vi "Write Param.vi"(0 "PID SP Limiter in":refnum<class "PID SP Limiter.lvclass">, 5 "SP_max":dbl=100.0 format="%.2f", 7 "SP_start_rate":dbl, 9 "SP_stop_rate":dbl, 12 "Out_H":dbl, 13 "Out_start_H":dbl, 14 "Out_stop_H":dbl) -> (4 "PID SP Limiter out":refnum<class "PID SP Limiter.lvclass">)   [LabVIEW 2019, in "control.lvlib" / "PID SP Limiter.lvclass"]
uses:
  PID SP Limiter.lvclass
  PID SP Limiter.lvclass/PID SP Limiter.ctl
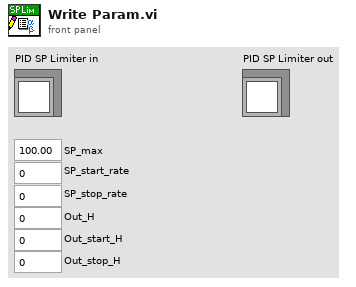
[diagram p1: front panel]
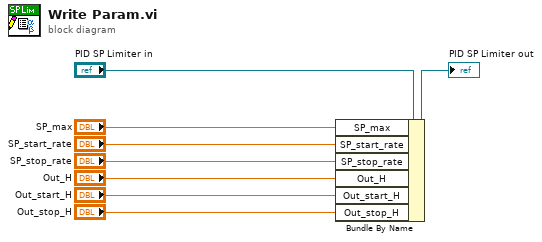
[diagram p0: block diagram]
diagram:
  n1 = Bundle By Name(cluster="PID SP Limiter in", "SP_max"="SP_max", "SP_start_rate"="SP_start_rate", "SP_stop_rate"="SP_stop_rate", "Out_H"="Out_H", "Out_start_H"="Out_start_H", "Out_stop_H"="Out_stop_H") -> (→"PID SP Limiter out":refnum<class "PID SP Limiter.lvclass">)
